vi "half adder.vi"() -> ()   [LabVIEW 2017]
panel:
  out "carry":bool
  out "sum":bool
  in  "B":bool
  in  "A":bool
  # "1"
  # "1"
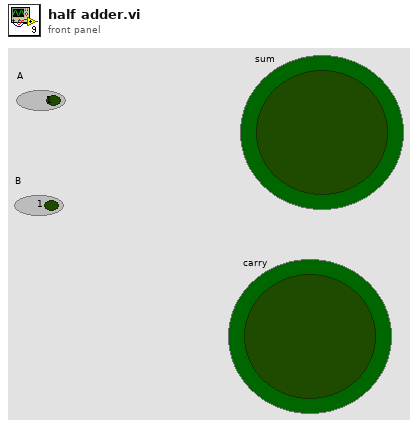
[diagram p1: front panel]
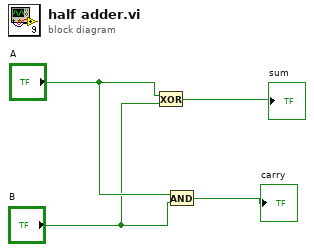
[diagram p0: block diagram]
diagram:
  n1 = Exclusive Or(1:"B", 2:"A") -> (0:→"sum":bool)
  n2 = And(x="A", y="B") -> (x .and. y?=→"carry":bool)
